vi "graficos2.vi"() -> ()   [LabVIEW 2019]
panel:
  out "Waveform Chart 2":dbl[](graph)
  out "Waveform Graph":dbl[](graph)
  out "Waveform Chart":dbl(graph)
  in  "stop":bool
  in  "Slide":dbl(slide) scale=0.0..50.0
  out "Thermometer":dbl(slide) scale=0.0..50.0
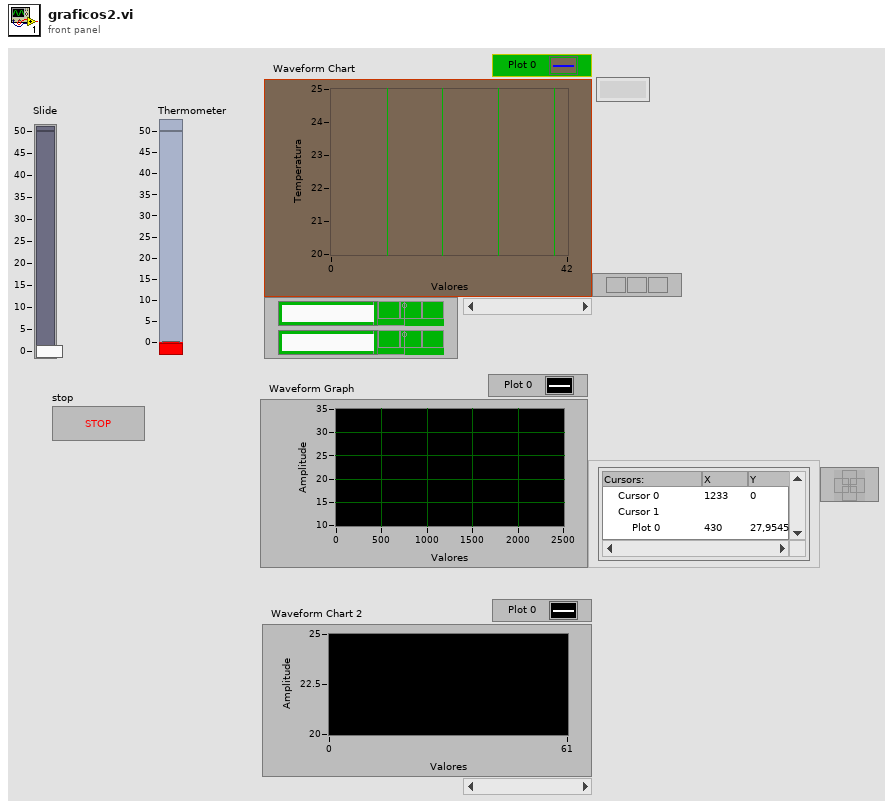
[diagram p1: front panel]
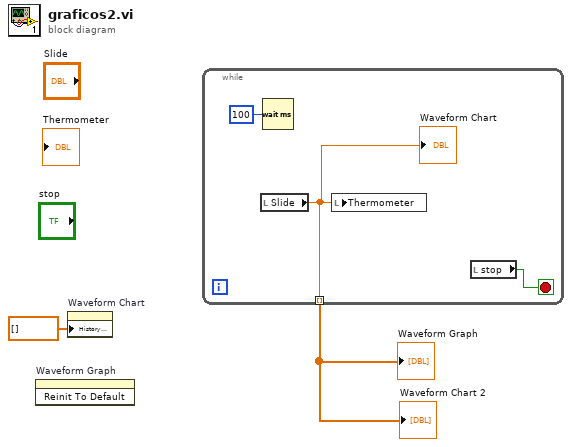
[diagram p0: block diagram]
diagram:
  n1 = invoke on="Waveform Graph" class="WFGraph (strict)" method="Reinit To Default"() -> ()  [unwired: 3 in, 3 out]
  n2 = property on="Waveform Chart" class="WFChart (strict)"("History Data"=dbl[] []) -> ()  [unwired: 2 in, 2 out]
  n3 = while {
    tunnel: [w3] -> w1 mode=indexing
    stop <- w4 stop-if-true
    n4 = local read "Slide"() -> (w3:dbl)
    "Waveform Chart" <- w3
    n5 = Wait (ms)(milliseconds to wait=u32 100) -> ()  [unwired: 1 out]
    n6 = local write "Thermometer"(w3) -> ()
    n7 = local read "stop"() -> (w4:bool)
  }
  "Waveform Graph" <- w1
  "Waveform Chart 2" <- w1
